vi "Modify Reference Control.vi"(8 "error in (no error)":errorcluster, 10 "Constructor Method VI in":refnum<vi>, 11 "QControl Creation in":refnum<class "QControl Creation.lvclass">) -> (0 "error out":errorcluster, 3 "QControl Creation (dup)":refnum<class "QControl Creation.lvclass">)   [LabVIEW 2015, in "QControl Creation.lvclass"]
doc: "<b> </b> <b> </b>\n©2016 Q Software Innovations, LLC (QSI)\nwritten by Quentin Alldredge\nproduced in LabVIEW 2015\n\nsupport@qsoftwareinnovations.com\nwww.qsoftwareinnovations.com\n\nAll rights reserved.\n\nRedistribution and use in source and binary forms, with or without modification, are permitted provided that the following conditions are met:\n\n * Redistributions of source code must retain the above copyright notice, this list of conditions and the following disclaimer.\n * Redistributions in binary form must reproduce the above copyright notice, this list of conditions and the following disclaimer in the documentation and/or other materials provided with the distribution.\n * Neither the name of Q Software Innovations, LLC. nor the names of its contributors may be used to endorse or promote products derived from this software without specific prior written permission.\n\nTHIS SOFTWARE IS PROVIDED BY THE COPYRIGHT HOLDERS AND CONTRIBUTORS \"AS IS\" AND ANY EXPRESS OR IMPLIED WARRANTIES, INCLUDING, BUT NOT LIMITED TO, THE IMPLIED WARRANTIES OF MERCHANTABILITY AND FITNESS FOR A PARTICULAR PURPOSE ARE DISCLAIMED. IN NO EVENT SHALL THE COPYRIGHT OWNER OR CONTRIBUTORS BE LIABLE FOR ANY DIRECT, INDIRECT, INCIDENTAL, SPECIAL, EXEMPLARY, OR CONSEQUENTIAL DAMAGES (INCLUDING, BUT NOT LIMITED TO, PROCUREMENT OF SUBSTITUTE GOODS OR SERVICES; LOSS OF USE, DATA, OR PROFITS; OR BUSINESS INTERRUPTION) HOWEVER CAUSED AND ON ANY THEORY OF LIABILITY, WHETHER IN CONTRACT, STRICT LIABILITY, OR TORT (INCLUDING NEGLIGENCE OR OTHERWISE) ARISING IN ANY WAY OUT OF THE USE OF THIS SOFTWARE, EVEN IF ADVISED OF THE POSSIBILITY OF SUCH DAMAGE."
uses:
  QControl Creation.lvclass
  <vilib>/Utility/traverseref.llb/TRef TravTarget.ctl
  QControl Creation.lvclass/QControl Creation.ctl
  <vilib>/Utility/error.llb/Error Cluster From Error Code.vi
  <vilib>/ErrorRing/Error Ring.xnode
  <vilib>/Utility/traverseref.llb/VI Scripting - Traverse.lvlib
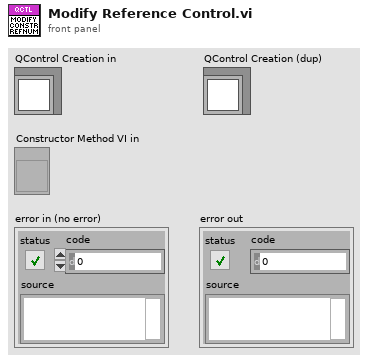
[diagram p1: front panel]
types:
  T1 = typedef "TRef TravTarget.ctl" = enum16{"FP", "BD", "Other"}
  T2 = typedef "LVPositionTypeDef.ctl" = cluster{"Left":i32, "Top":i32}
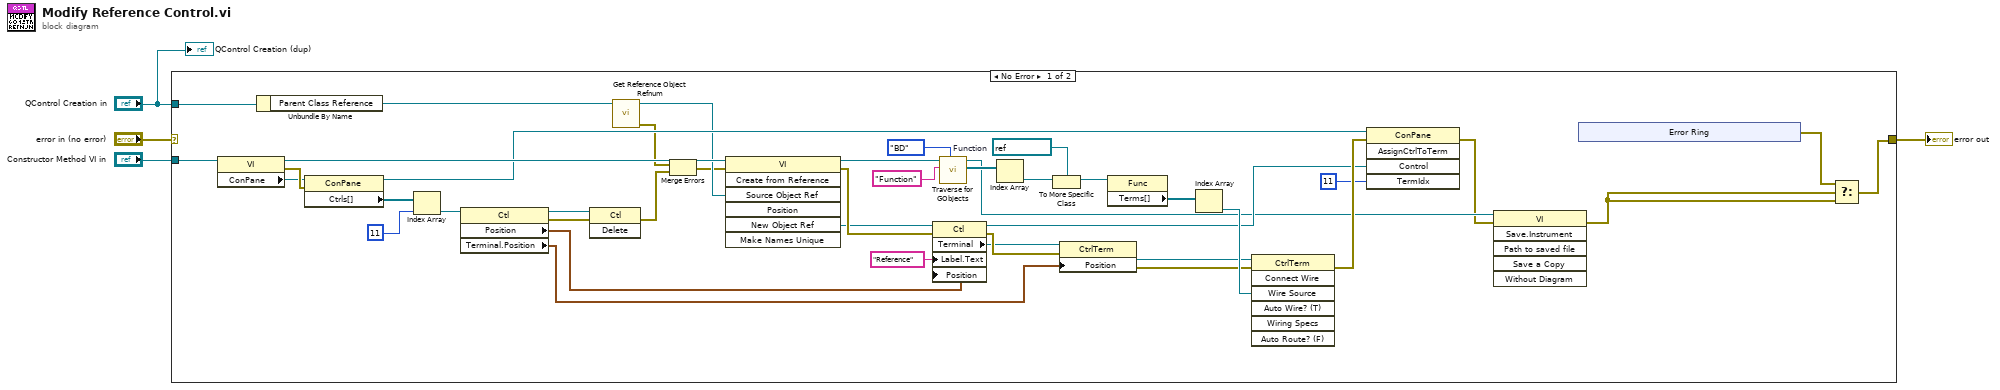
[diagram p0: block diagram]
diagram:
  n1 = case shown="No Error" "error in (no error)" {
    selector: "error in (no error)" -> [_ w52]
    tunnel: "QControl Creation in" -> [w45 _]
    tunnel: [w5 w52] -> w4
    tunnel: "Constructor Method VI in" -> [w44 _]
    frame No Error {
      w37 = refnum<vi> refnum  # Function
      n2 = property class="VI"(reference=w44) -> (reference out=w43:refnum<vi>, error out=w13:errorcluster, "ConPane"=w12:refnum<vi>)  [unwired: 1 in]
      n3 = Unbundle By Name(w45) -> ("Parent Class Reference"=w46:refnum<vi>)
      n4 = property class="ConPane"(reference=w12, error in=w13) -> (reference out=w20:refnum<vi>, "Ctrls[]"=w14:refnum<vi>[])  [unwired: 1 out]
      n5 = Index Array(array=w14, index=11) -> (element=w17:refnum<vi>)
      n6 = property class="Ctl"(reference=w17) -> (reference out=w19:refnum<vi>, error out=w42:errorcluster, "Position"=w41:T2, "Terminal.Position"=w27:T2)  [unwired: 1 in]
      n7 = invoke class="Ctl" method="Delete"(reference=w19, error in=w42) -> (error out=w29:errorcluster)  [unwired: 1 in, 2 out]
      n8 = call "Get Reference Object Refnum.vi"("LVClassLibrary in"=w46) -> ("error out"=w10:errorcluster, "LVObjectRefNum out"=w16:refnum<vi>)  [unwired: 8 in, 1 out]
      n9 = Merge Errors(w10, w29) -> (w11:errorcluster)
      n10 = invoke class="VI" method="Create from Reference"(reference=w43, error in=w11, "Source Object Ref"=w16) -> (reference out=w32:refnum<vi>, error out=w30:errorcluster, "New Object Ref"=w18:refnum<vi>)  [unwired: 4 in, 4 out]
      n11 = property class="Ctl"(reference=w18, error in=w30, "Label.Text"="Reference", "Position"=w41) -> (reference out=w21:refnum<vi>, error out=w31:errorcluster, "Terminal"=w25:refnum<vi>)
      n12 = call <vilib>:"Traverse for GObjects.vi"("Traverse Target"=TRef_TravTarget."BD", "Class Name"="Function" ("Label.Text"), "VI Refnum"=w32) -> ("References"=w35:refnum<vi>[], "dup VI Refnum"=w9:refnum<vi>)  [unwired: 5 in, 2 out]
      n13 = Index Array(array=w35) -> (element=w36:refnum<vi>)  [unwired: 1 in]
      n14 = To More Specific Class(target class=w37, reference=w36) -> (specific class reference=w38:refnum<vi>)  [unwired: 1 in, 1 out]
      n15 = property class="CtrlTerm"(reference=w25, error in=w31, "Position"=w27) -> (reference out=w26:refnum<vi>, error out=w24:errorcluster)
      n16 = property class="Func"(reference=w38) -> ("Terms[]"=w39:refnum<vi>[])  [unwired: 1 in, 2 out]
      n17 = Index Array(array=w39) -> (element=w40:refnum<vi>)  [unwired: 1 in]
      n18 = invoke class="CtrlTerm" method="Connect Wire"(reference=w26, error in=w24, "Wire Source"=w40) -> (error out=w23:errorcluster)  [unwired: 4 in, 6 out]
      n19 = invoke class="ConPane" method="AssignCtrlToTerm"(reference=w20, error in=w23, "Control"=w21, "TermIdx"=u32 11 ("Terminal Index")) -> (error out=w8:errorcluster)  [unwired: 1 in, 4 out]
      n20 = invoke class="VI" method="Save.Instrument"(reference=w9, error in=w8) -> (error out=w7:errorcluster)  [unwired: 4 in, 5 out]
      n21 = xnode "Error Ring"() -> ("error out"=w6:errorcluster)
      n22 = Select(t=w6, s=w7, f=w7) -> (s? t:f=w5:errorcluster)
    }
    frame Error {
    }
  }
  "error out" <- w4
  "QControl Creation (dup)" <- "QControl Creation in"
